vi "resistivity_measurement.vi"(0 "S-l Ratio":dbl, 2 "General Time":dbl, 3 "Measurement Data 1":dbl[](array[numeric]), 4 "Measurement Data 2":dbl[](array[numeric])) -> (5 "Data Out":dbl[](array[numeric]), 6 "Resistivity Graph":cluster{"Y":dbl[], "Y":dbl[]}[](graph))   [LabVIEW 2011]
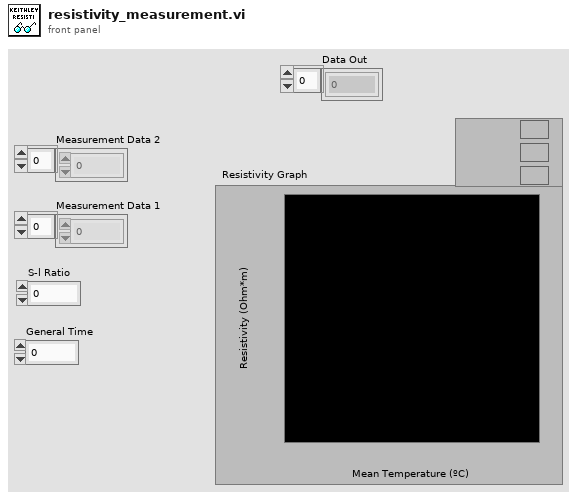
[diagram p1: front panel]
types:
  T1 = cluster{"Data Keithley Out[0]":dbl, "Data Keithley Out[1]":dbl, "Data Keithley Out[2]":dbl, "Data Keithley Out[3]":dbl, "Data Keithley Out[4]":dbl, "Data Keithley Out[5]":dbl, "Data Keithley Out[6]":dbl, "Data Keithley Out[7]":dbl, "Data Keithley Out[8]":dbl}
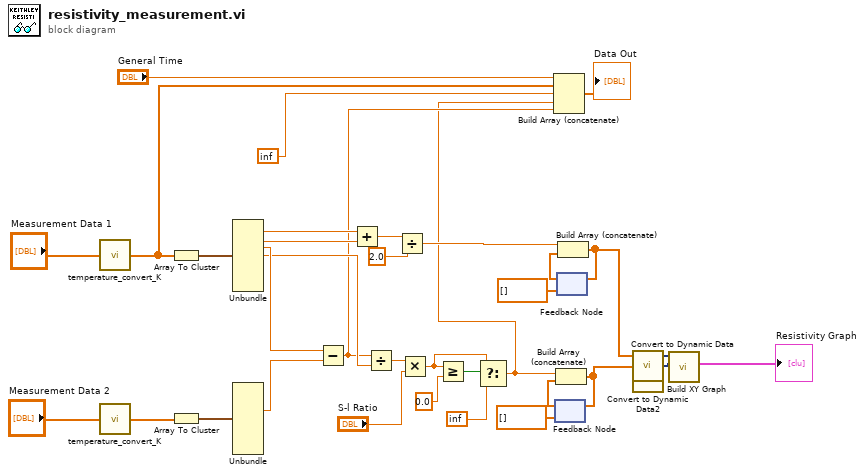
[diagram p0: block diagram]
diagram:
  n1 = call "temperature_convert_K.vi"("Data Keithley In"="Measurement Data 1") -> ("Data Keithley Out"=w12:dbl[])  [unwired: 4 in]
  n2 = call "temperature_convert_K.vi"("Data Keithley In"="Measurement Data 2") -> ("Data Keithley Out"=w11:dbl[])  [unwired: 4 in]
  n3 = Array To Cluster(array=w12) -> (cluster=w34:T1)
  n4 = Array To Cluster(array=w11) -> (cluster=w31:T1)
  n5 = Unbundle(w34) -> ("Data Keithley Out[1]"=w28:dbl, "Data Keithley Out[2]"=w27:dbl, "Data Keithley Out[3]"=w30:dbl, "Data Keithley Out[4]"=w29:dbl)  [unwired: 5 out]
  n6 = Unbundle(w31) -> ("Data Keithley Out[3]"=w13:dbl)  [unwired: 8 out]
  n7 = Subtract(x=w30, y=w13) -> (x-y=w7:dbl)
  n8 = Add(x=w28, y=w27) -> (x+y=w26:dbl)
  n9 = Divide(x=w7, y=w29) -> (x/y=w15:dbl)
  n10 = Divide(x=w26, y=2.0) -> (x/y=w8:dbl)
  n11 = Multiply(x=w15, y="S-l Ratio") -> (x*y=w4:dbl)
  n12 = Greater Or Equal?(x=w4, y=0.0) -> (x >= y?=w5:bool)
  n13 = Select(t=w4, s=w5, f=inf) -> (s? t:f=w1:dbl)
  n14 = Build Array (concatenate)("General Time", w12, inf, w1, w7) -> (→"Data Out":dbl[])
  n15 = feedback #1(dbl[] []) -> (w24:dbl[])
  n16 = Build Array (concatenate)(w1, w24) -> (w17:dbl[])
  n17 = feedback-in #1(w17) -> ()
  n18 = feedback #2(dbl[] []) -> (w22:dbl[])
  n19 = Build Array (concatenate)(w8, w22) -> (w19:dbl[])
  n20 = feedback-in #2(w19) -> ()
  n21 = call "Convert to Dynamic Data"("Array"=w19) -> ("Dynamic Data Type"=w18:dynamicdata)  [unwired: 3 in]
  n22 = call "Convert to Dynamic Data2"("Array"=w17) -> ("Dynamic Data Type"=w16:dynamicdata)  [unwired: 3 in]
  n23 = call "Build XY Graph"("Y Input"=w16, "X Input"=w18) -> ("XY Graph"=→"Resistivity Graph":cluster{"Y":dbl[], "Y":dbl[]}[])  [unwired: 3 in, 6 out]
